vi "User Events - Get.vi"(8 "error in":errorcluster) -> (0 "error out":errorcluster, 3 "User Events Cluster":T1)   [LabVIEW 2024, in "User Events.lvlib"]
uses:
  User Events.lvlib
  General Type Defs/User Events Cluster.ctl
  General Type Defs/FGV States.ctl
  General Type Defs/General Type Defs.lvlib
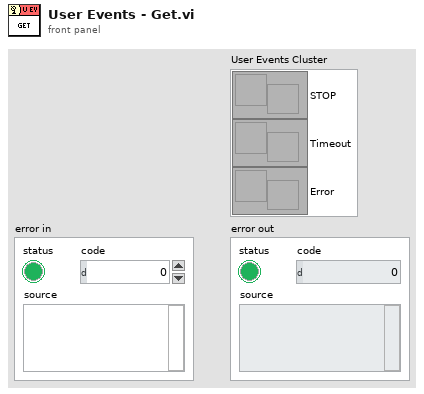
[diagram p1: front panel]
types:
  T1 = typedef "General Type Defs.lvlib/User Events Cluster.ctl" = cluster{"STOP":refnum<user-event>, "Timeout":refnum<user-event>, "Error":refnum<user-event>}
  T2 = typedef "General Type Defs.lvlib/FGV States.ctl" = enum16{"Create", "Get", "Destroy"}
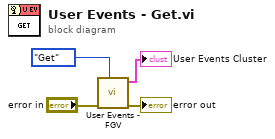
[diagram p0: block diagram]
diagram:
  n1 = call "User Events - FGV.vi"("FGV States"=FGV_States."Get", "error in"="error in") -> ("error out"=→"error out":errorcluster, "User Events Cluster"=→"User Events Cluster":T1)  [unwired: 8 in]
